vi "PH_Beckhoff.read and write Hardware.vi"(0 "i ref in":refnum<vi>, 1 "Klemmencluster: # of":T1, 2 "Beckhoff Access":T2, 3 "Current Values":T3, 5 "error in":errorcluster) -> (11 "Current Digital Output":bool[](array[boolean]), 13 "Current Digital Inputs":bool[](array[boolean]), 14 "i ref out":refnum<vi>, 15 "Current Sonderklemmen  Inputs":u64[](array[numeric]), 16 "Current Analog Inputs":u32[](array[numeric]), 17 "Current Analog Outputs":u32[](array[numeric]), 18 "Read and write successful?":bool, 19 "error out":errorcluster)   [LabVIEW 2014, in "PH_Beckhoff.lvlib"]
doc: "This VI communicates with the hardware to get the current values and to set the wanted values."
uses:
  PH_Beckhoff.lvlib
  PH_Beckhoff.Values.ctl
  PH_Beckhoff.Sonderklemmen Inputs.ctl
  PH_Beckhoff.Analog Inputs.ctl
  PH_Beckhoff.Scaling Type.ctl
  PH_Beckhoff.Analog Outputs.ctl
  PH_Beckhoff.Digital Inputs.ctl
  PH_Beckhoff.Digital Outputs.ctl
  non_GPL/instr.lib/Beckhoff/Helpers/Beckhoff Access.ctl
  non_GPL/instr.lib/Beckhoff/Helpers/Klemmendeclarer.ctl
  non_GPL/instr.lib/Beckhoff/Beckhoff - Driver np.lvlib
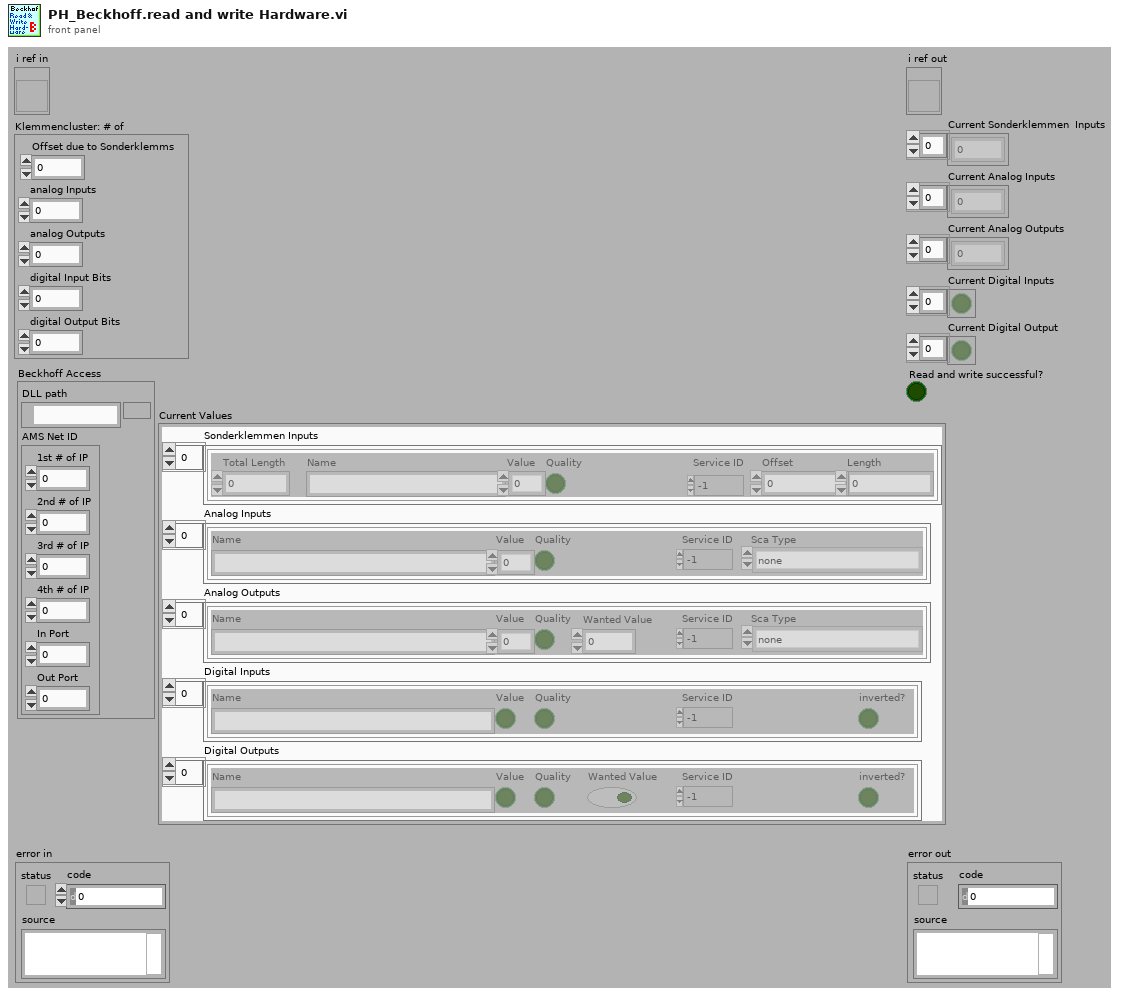
[diagram p1: front panel]
types:
  T1 = typedef "Beckhoff - Driver np.lvlib/Klemmendeclarer.ctl" = cluster{"Offset due to Sonderklemms":u32, "analog Inputs":u32, "analog Outputs":u32, "digital Input Bits":u32, "digital Output Bits":u32}
  T2 = typedef "Beckhoff - Driver np.lvlib/Beckhoff Access.ctl" = cluster{"DLL path":path, "AMS Net ID":cluster{"1st # of IP":u8, "2nd # of IP":u8, "3rd # of IP":u8, "4th # of IP":u8, "In Port":u8, "Out Port":u8}}
  T3 = typedef "PH_Beckhoff.lvlib/PH_Beckhoff.Values.ctl" = cluster{"Sonderklemmen Inputs":T4, "Analog Inputs":T5, "Analog Outputs":T7, "Digital Inputs":T8, "Digital Outputs":T9}
  T4 = typedef "PH_Beckhoff.lvlib/PH_Beckhoff.Sonderklemmen Inputs.ctl" = cluster{"Total Length":u32, "Name":string, "Value":u64, "Quality":bool, "Service ID":i32, "Offset":u32, "Length":u32}[]
  T5 = typedef "PH_Beckhoff.lvlib/PH_Beckhoff.Analog Inputs.ctl" = cluster{"Name":string, "Value":u32, "Quality":bool, "Service ID":i32, "Sca Type":T6}[]
  T6 = typedef "PH_Beckhoff.lvlib/PH_Beckhoff.Scaling Type.ctl" = enum16{"none", "0 ... 15 Bit -> 0 ... 5", "0 ... 15 Bit -> 0 ... 10", "0 ... 15 Bit -> 0 ... 25", "0 ... 15 Bit -> 4 ... 20", "0 ... 15 Bit -> 0 ... 1", "0 ... 15 Bit -> 0 ... 20000", "0 ... 15 Bit -> 0 ... 24000"}
  T7 = typedef "PH_Beckhoff.lvlib/PH_Beckhoff.Analog Outputs.ctl" = cluster{"Name":string, "Value":u32, "Quality":bool, "Wanted Value":u32, "Service ID":i32, "Sca Type":T6}[]
  T8 = typedef "PH_Beckhoff.lvlib/PH_Beckhoff.Digital Inputs.ctl" = cluster{"Name":string, "Value":bool, "Quality":bool, "Service ID":i32, "inverted?":bool}[]
  T9 = typedef "PH_Beckhoff.lvlib/PH_Beckhoff.Digital Outputs.ctl" = cluster{"Name":string, "Value":bool, "Quality":bool, "Wanted Value":bool, "Service ID":i32, "inverted?":bool}[]
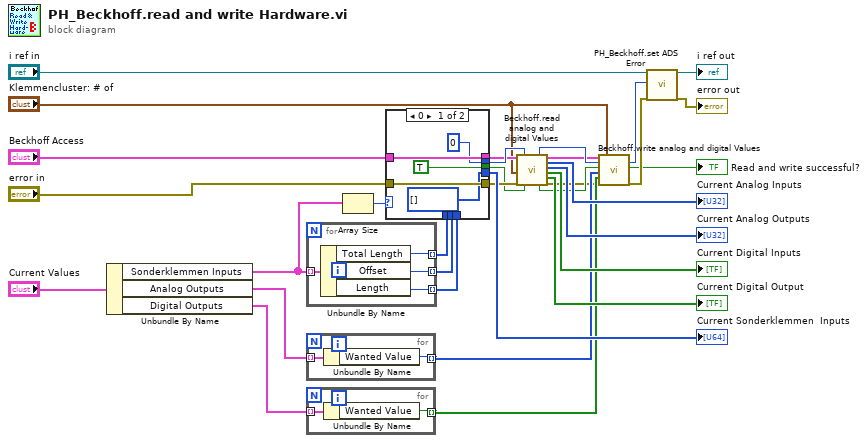
[diagram p0: block diagram]
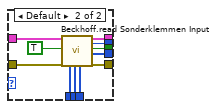
[diagram p2: hidden frame]
diagram:
  n1 = Unbundle By Name("Current Values") -> ("Sonderklemmen Inputs"=w30:T4, "Analog Outputs"=w31:T7, "Digital Outputs"=w32:T9)
  n2 = for {
    tunnel: w30 -> [w36] mode=indexing
    tunnel: [w35] -> w24 mode=indexing
    tunnel: [w34] -> w25 mode=indexing
    tunnel: [w33] -> w26 mode=indexing
    n3 = Unbundle By Name(w36) -> ("Total Length"=w35:u32, "Offset"=w34:u32, "Length"=w33:u32)
  }
  n4 = for {
    tunnel: w31 -> [w38] mode=indexing
    tunnel: [w37] -> w10 mode=indexing
    n5 = Unbundle By Name(w38) -> ("Wanted Value"=w37:u32)
  }
  n6 = for {
    tunnel: w32 -> [w40] mode=indexing
    tunnel: [w39] -> w9 mode=indexing
    n7 = Unbundle By Name(w40) -> ("Wanted Value"=w39:bool)
  }
  n8 = Array Size(array=w30) -> (size(s)=w28:i32)
  n9 = case shown="0" w28 {
    tunnel: "Beckhoff Access" -> [w45 w56]
    tunnel: [w45 w55] -> w19
    tunnel: [0 ("ADS Error out") w54] -> w20
    tunnel: [TRUE ("read successful?") w53] -> w21
    tunnel: [w44 w52] -> w22
    tunnel: "error in" -> [w44 w51]
    tunnel: w24 -> [_ w50]
    tunnel: w25 -> [_ w49]
    tunnel: w26 -> [_ w48]
    tunnel: [u64[] [] ("Current Sonderklemmen  Inputs") w47] -> w27
    frame 0 {
    }
    frame Default {
      n10 = call "Beckhoff.read Sonderklemmen Input.vi"("AMS Net ID in"=w56, "Read?"=TRUE, "error in"=w51, "Total Lengths"=w50, "Offsets"=w49, "Lengths"=w48) -> ("AMS Net ID out"=w55:T2, "ADS Error out"=w54:i32, "read successful?"=w53:bool, "Current Sonderklemmen  Inputs"=w47:u64[], "error out"=w52:errorcluster)  [unwired: 9 in]
    }
  }
  "Current Sonderklemmen  Inputs" <- w27
  n11 = call "Beckhoff.read analog and digital Values.vi"("AMS Net ID in"=w19, "Klemmendeclarer: # of"="Klemmencluster: # of", "error in"=w22, "ADS Error in (0)"=w20, "Read?"=w21) -> ("ADS Error out"=w3:i32, "read successful?"=w5:bool, "AMS Net ID out"=w2:T2, "Current Analog Inputs"=→"Current Analog Inputs":u32[], "Current Analog Outputs"=→"Current Analog Outputs":u32[], "Current Digital Inputs"=→"Current Digital Inputs":bool[], "Current Digital Output"=→"Current Digital Output":bool[], "error out"=w4:errorcluster)  [unwired: 7 in]
  n12 = call "Beckhoff.write analog and digital Values.vi"("AMS Net ID in"=w2, "ADS Error in (0)"=w3, "Write?"=w5, "Analog Outputs to be set"=w10, "Digital Outputs to be set"=w9, "error in"=w4, "Klemmedeclarer: # of ..."="Klemmencluster: # of") -> ("ADS Error out"=w6:i32, "write successful?"=→"Read and write successful?":bool, "error out"=w8:errorcluster)  [unwired: 9 in, 1 out]
  n13 = call "PH_Beckhoff.set ADS Error.vi"("i ref in"="i ref in", "ADS Error"=w6, "error in"=w8) -> ("i ref out"=→"i ref out":refnum<vi>, "error out"=→"error out":errorcluster)  [unwired: 15 in]
